vi "Evaluate U and V from calib polysurf.vi"(2 "alpha(rad) coeffs":dbl[](array[numeric])=[-6.408819091280157, -77.31287064703562, 39.596088887046406, -13.655557326518679, 92.22252547020423, -0.3836387160655101, 20.987115315584187, -49.60347017734866, -22.12520782591642, 17.137886389734525], 3 "E1 / G1 + O1":dbl=2.3, 4 "Ucal coeffs":dbl[](array[numeric])=[-145.45710480983897, 100.50457508854375, -59.6837287964547, 9.197373198480307, 113.85234870232155, 21.356403852079225, 1.852404482942991, -70.69389530720044, -6.371778227926893, 14.525514681706548], 5 "cap indicial sum to n":bool=TRUE, 6 "surface order (n)":i32=3, 7 "E2 / G2 + O2":dbl=2.6) -> (0 "V (m/s)":dbl=-1.8332814538592657 format="%.6f", 1 "U (m/s)":dbl=7.542490254728585 format="%.6f")   [LabVIEW 2011]
uses:
  <vilib>/Analysis/baseanly.llb/Real Dot Product.vi
  <vilib>/Analysis/NI_AALBase.lvlib
panel:
  # "Paul Nathan 02/02/10"
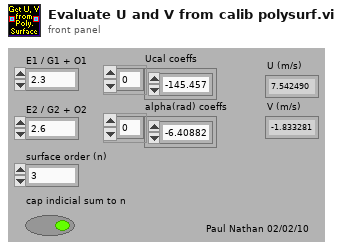
[diagram p1: front panel]
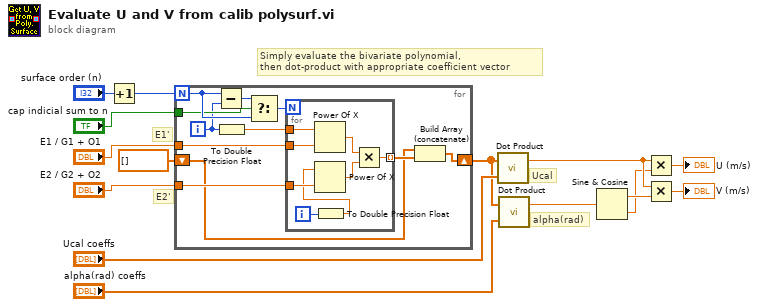
[diagram p0: block diagram]
diagram:
  # "Simply evaluate the bivariate polynomial,\nthen dot-product with appropriate coefficient vector"
  # "alpha(rad)"
  # "Ucal"
  # "E2'"
  # "E1'"
  n1 = Increment(x="surface order (n)") -> (x+1=w13:i32)
  n2 = for {
    N: w13 -> [w25]
    tunnel: "cap indicial sum to n" -> [w24]
    tunnel: "E1 / G1 + O1" -> [w22]
    tunnel: "E2 / G2 + O2" -> [w21]
    shift-right: [w17] -> w8
    shift-left: dbl[] [] -> [w16]
    i -> [w20]
    n3 = Subtract(x=w25, y=w20) -> (x-y=w26:i32)
    n4 = To Double Precision Float(number=w20) -> (double precision float=w19:dbl)
    n5 = Select(t=w26, s=w24, f=w25) -> (s? t:f=w23:i32)
    n6 = for {
      N: w23 -> [_]
      tunnel: w22 -> [w32]
      tunnel: w21 -> [w31]
      tunnel: w19 -> [w33]
      tunnel: [w27] -> w18 mode=indexing
      i -> [w34]
      # "j"
      n7 = Power Of X(1:w32, 2:w33) -> (0:w30:dbl)
      n8 = To Double Precision Float(number=w34) -> (double precision float=w28:dbl)
      n9 = Power Of X(1:w31, 2:w28) -> (0:w29:dbl)
      n10 = Multiply(x=w30, y=w29) -> (x*y=w27:dbl)
    }
    n11 = Build Array (concatenate)(w16, w18) -> (w17:dbl[])
  }
  n12 = call-poly <vilib>:"Dot Product.vi"("Y Vector"="Ucal coeffs", "X Vector"=w8) -> ("X * Y"=w3:dbl)  [unwired: 1 out]
  n13 = call-poly <vilib>:"Dot Product.vi"("Y Vector"="alpha(rad) coeffs", "X Vector"=w8) -> ("X * Y"=w6:dbl)  [unwired: 1 out]
  n14 = Sine & Cosine(0:w6) -> (1:w2:dbl, 2:w1:dbl)
  n15 = Multiply(x=w3, y=w1) -> (x*y=→"U (m/s)":dbl)
  n16 = Multiply(x=w3, y=w2) -> (x*y=→"V (m/s)":dbl)
